vi "FlpLib AlphaBetaToABC_UnitaryMagnitude 2.vi"(0 "alpha":sgl, 5 "beta":sgl) -> (4 "A":sgl, 6 "B":sgl, 8 "C":sgl)   [LabVIEW 2017]
uses:
  <userlib>/_NI FLP Library/FPGA/outsideSCTL/FlpLib Multiply Shared Instance 2.vi
  <userlib>/_NI FLP Library/FPGA/outsideSCTL/FlpLib Subtract Shared Instance 2.vi
  <userlib>/_NI FLP Library/FPGA/outsideSCTL/FlpLib Add Shared Instance 2.vi
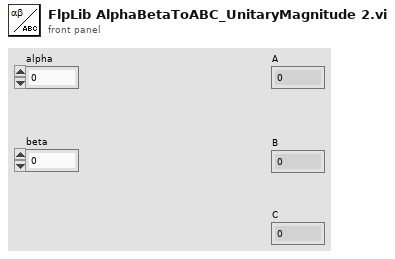
[diagram p1: front panel]
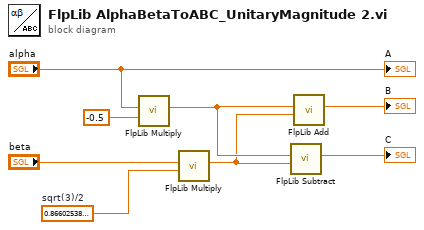
[diagram p0: block diagram]
diagram:
  w1 = sgl 0.8660254  # sqrt(3)/2
  n1 = call-poly <userlib>:"FlpLib Multiply.vi"("y"=sgl -0.5, "x"="alpha") -> ("x*y"=w7:sgl)  [unwired: 5 in]
  n2 = call-poly <userlib>:"FlpLib Multiply.vi"("y"=w1, "x"="beta") -> ("x*y"=w6:sgl)  [unwired: 5 in]
  n3 = call-poly <userlib>:"FlpLib Subtract.vi"("y"=w6, "x"=w7) -> ("x-y"=→"C":sgl)  [unwired: 5 in]
  n4 = call-poly <userlib>:"FlpLib Add.vi"("y"=w6, "x"=w7) -> ("x+y"=→"B":sgl)  [unwired: 5 in]
  "A" <- "alpha"
